vi "Andor Ixon_Settings.vi"() -> ()   [LabVIEW 2012]
uses:
  <userlib>/atmcd64d.llb/HSSpeed_type typedef.ctl
panel:
  in  "OK Button":bool
  in  "Vertical clock voltage":i32(ring) items=["Normal", "+1", "+2", "+3", "+4"]
  in  "Shift speed":i32(ring) items=["0.564720", "1.016496", "1.920048", "[3.727152]"]
  in  "Readout rate":i32(ring) items=["35.00MHz", "27.00MHz", "13.00MHz"]
  in  "Pre-amplifier gain":i32(ring) items=["1.000000x", "1.900000x", "3.700000x"]
  in  "Binning":i32[](array[numeric])
  in  "ROI":i32[][](array[numeric])
  in  "EM Gain":i32 min=3
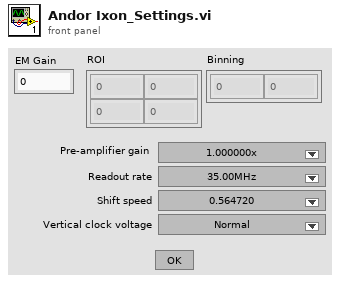
[diagram p1: front panel]
types:
  T1 = typedef "HSSpeed_type typedef.ctl" = enum16{"EM Amp", "Conventional Amp"}
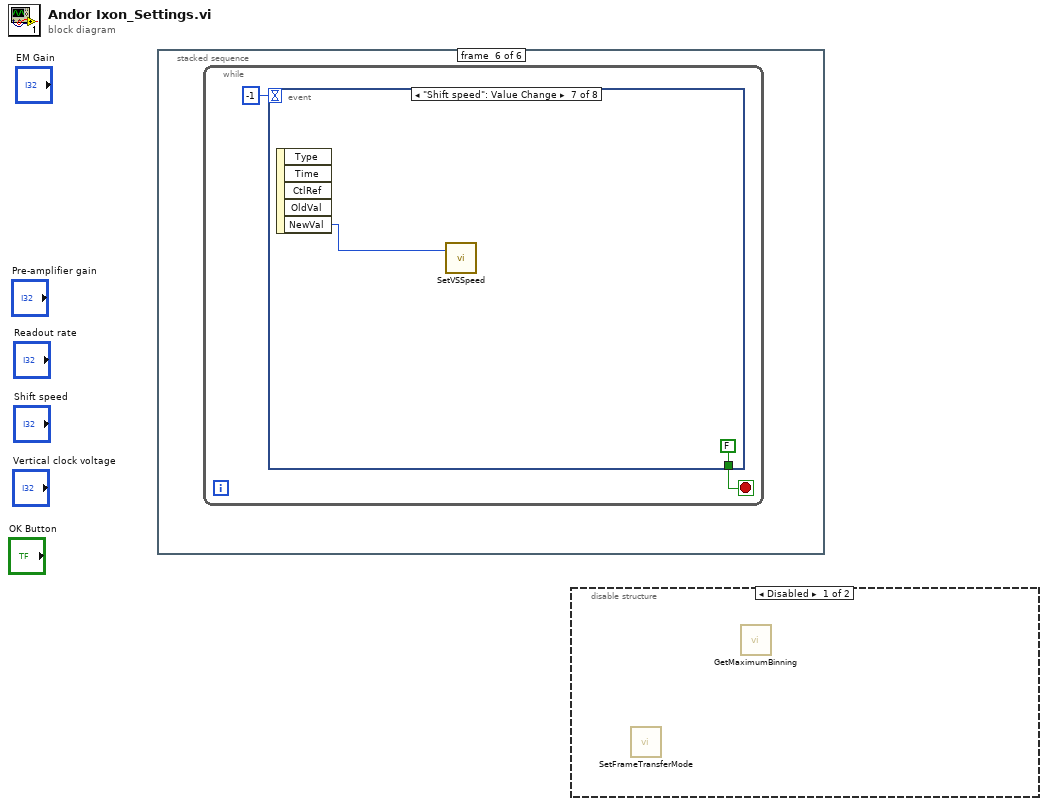
[diagram p0: block diagram]
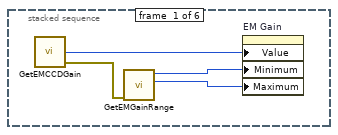
[diagram p3: hidden frame]
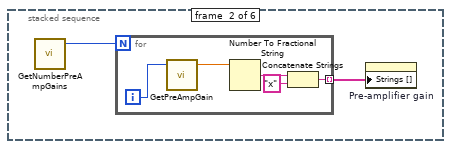
[diagram p4: hidden frame]
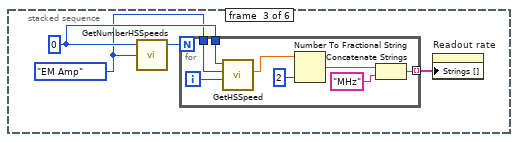
[diagram p5: hidden frame]
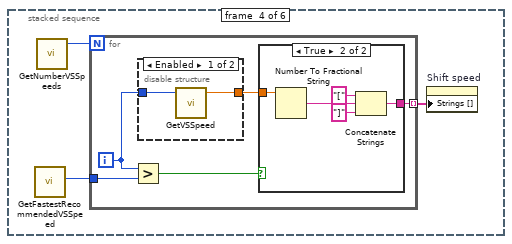
[diagram p6: hidden frame]
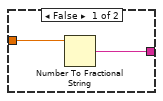
[diagram p7: hidden frame]
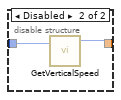
[diagram p8: hidden frame]
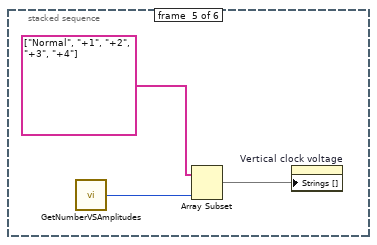
[diagram p9: hidden frame]
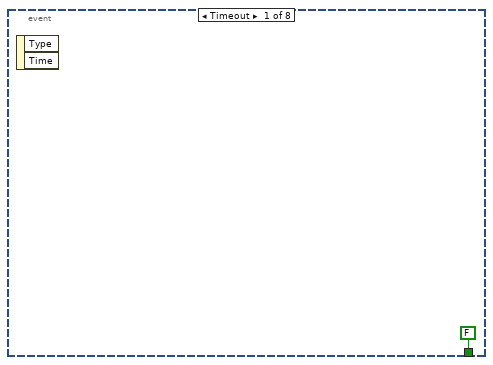
[diagram p10: hidden frame]
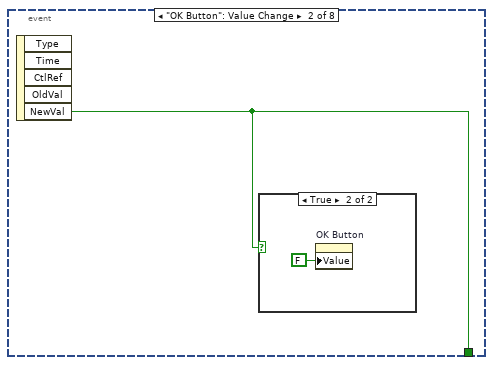
[diagram p11: hidden frame]
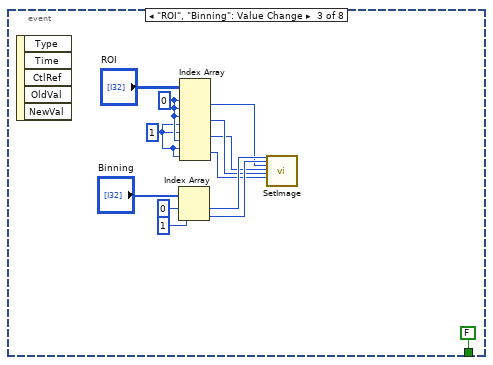
[diagram p13: hidden frame]
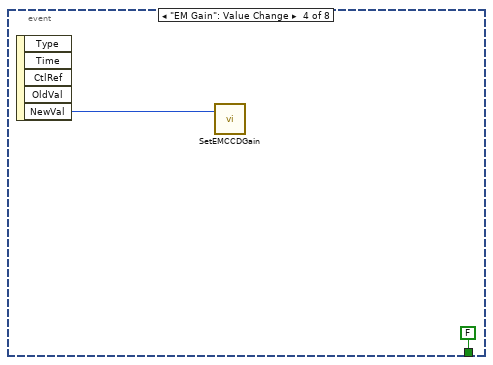
[diagram p14: hidden frame]
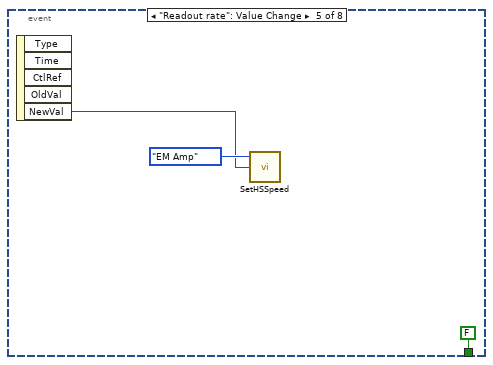
[diagram p15: hidden frame]
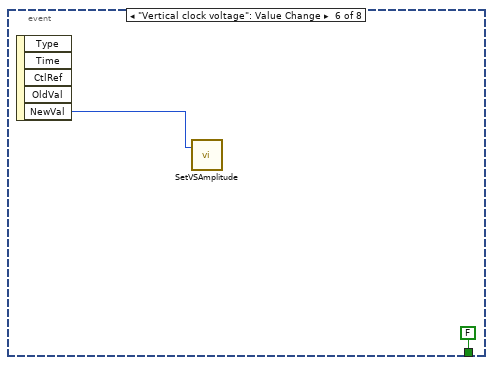
[diagram p16: hidden frame]
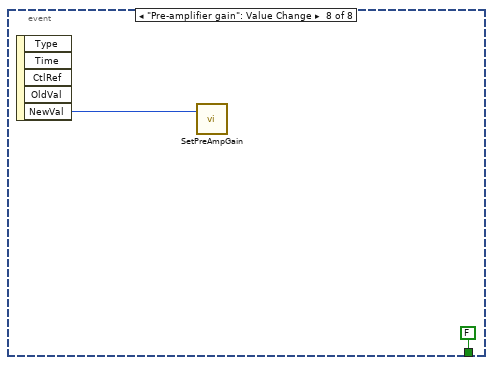
[diagram p17: hidden frame]
diagram:
  n1 = stacked-sequence {
    frame #0 {
      n2 = call <userlib>:"GetEMCCDGain.vi"() -> ("error out"=w1:errorcluster, "gain"=w4:u32)  [unwired: 3 in, 1 out]
      n3 = call <userlib>:"GetEMGainRange.vi"("error in (no error)"=w1) -> ("high"=w2:i32, "low"=w3:i32)  [unwired: 3 in, 2 out]
      n4 = property on="EM Gain" class="DigNum (strict)"("Value"=w4, "Minimum"=w3, "Maximum"=w2) -> ()  [unwired: 2 in, 2 out]
    }
    frame #1 {
      n5 = call <userlib>:"GetNumberPreAmpGains.vi"() -> ("number"=w5:i32)  [unwired: 3 in, 2 out]
      n6 = for {
        N: w5 -> [_]
        tunnel: [w9] -> w6 mode=indexing
        i -> [w8]
        n7 = call <userlib>:"GetPreAmpGain.vi"("index"=w8) -> ("gain"=w7:sgl)  [unwired: 2 in, 2 out]
        n8 = Number To Fractional String(number=w7) -> (F-format string=w11:string)  [unwired: 3 in]
        n9 = Concatenate Strings(w11, "x" ("string")) -> (w9:string)
      }
      n10 = property on="Pre-amplifier gain" class="Ring (strict)"("Strings []"=w6) -> ()  [unwired: 2 in, 2 out]
    }
    frame #2 {
      w12 = HSSpeed_type_typedef."EM Amp" ("type")
      w13 = 0 ("channel")
      n11 = call <userlib>:"GetNumberHSSpeeds.vi"("type"=w12, "channel"=w13) -> ("number"=w14:i32)  [unwired: 1 in, 2 out]
      n12 = for {
        N: w14 -> [_]
        tunnel: [w21] -> w15 mode=indexing
        tunnel: w13 -> [w18]
        tunnel: w12 -> [w17]
        i -> [w19]
        n13 = call <userlib>:"GetHSSpeed.vi"("index"=w19, "type"=w17, "channel"=w18) -> ("speed"=w20:sgl)  [unwired: 2 in, 2 out]
        n14 = Number To Fractional String(number=w20, precision (6)=i16 2) -> (F-format string=w23:string)  [unwired: 2 in]
        n15 = Concatenate Strings(w23, "MHz" ("string")) -> (w21:string)
      }
      n16 = property on="Readout rate" class="Ring (strict)"("Strings []"=w15) -> ()  [unwired: 2 in, 2 out]
    }
    frame #3 {
      n17 = call <userlib>:"GetFastestRecommendedVSSpeed.vi"() -> ("index"=w24:u32)  [unwired: 4 in, 3 out]
      n18 = call <userlib>:"GetNumberVSSpeeds.vi"() -> ("number"=w25:i32)  [unwired: 3 in, 2 out]
      n19 = for {
        N: w25 -> [_]
        tunnel: [w30] -> w26 mode=indexing
        tunnel: w24 -> [w28]
        i -> [w29]
        n20 = Greater?(x=w29, y=w28) -> (0:w27:bool)
        n21 = disable-structure shown="Enabled" {
          disable-tunnel: [w39 w41] -> w31
          disable-tunnel: w29 -> [w40 w42]
          frame Enabled {
            n22 = call <userlib>:"GetVSSpeed.vi"("index"=w40) -> ("speed"=w39:sgl)  [unwired: 2 in, 2 out]
          }
          frame Disabled {
            n23 = call <userlib>:"GetVerticalSpeed.vi"("index"=w42) -> ("speed"=w41:i32)  [unwired: 1 in, 2 out]
          }
        }
        n24 = case shown="True" w27 {
          tunnel: w31 -> [w33 w38]
          tunnel: [w32 w36] -> w30
          frame False {
            n25 = Number To Fractional String(number=w33) -> (F-format string=w32:string)  [unwired: 3 in]
          }
          frame True {
            n26 = Number To Fractional String(number=w38) -> (F-format string=w37:string)  [unwired: 3 in]
            n27 = Concatenate Strings("[" ("string"), w37, "]" ("string")) -> (w36:string)
          }
        }
      }
      n28 = property on="Shift speed" class="Ring (strict)"("Strings []"=w26) -> ()  [unwired: 2 in, 2 out]
    }
    frame #4 {
      n29 = call <userlib>:"GetNumberVSAmplitudes.vi"() -> ("number"=w43:i32)  [unwired: 3 in, 2 out]
      n30 = Array Subset(array=string[] ["Normal", "+1", "+2", "+3", "+4"], length=w43) -> (w44:string[])  [unwired: 1 in]
      n31 = property on="Vertical clock voltage" class="Ring (strict)"("Strings []"=w44) -> ()  [unwired: 2 in, 2 out]
    }
    frame #5 {
      n32 = while {
        stop <- w46 stop-if-true
        n33 = event shown="[6] \"Shift speed\": Value Change" {
          selector: _ -> [_ _ _ _ _ _ _ _]
          dyn-events: _ -> [_ _ _ _ _ _ _ _]
          timeout: -1 -> [_ _ _ _ _ _ _ _]
          tunnel: [FALSE ("NewVal") w49 FALSE ("NewVal") FALSE ("NewVal") FALSE ("NewVal") FALSE ("NewVal") FALSE ("NewVal") FALSE ("NewVal")] -> w46
          event Timeout {
            n34 = event-data() -> ()  [unwired: 1 in, 2 out]
          }
          event "OK Button": Value Change {
            n35 = event-data() -> ("NewVal"=w49:bool)  [unwired: 1 in, 4 out]
            n36 = case shown="True" w49 {
              frame False {
              }
              frame True {
                n37 = property on="OK Button" class="Bool (strict)"("Value"=FALSE ("OK Button")) -> ()  [unwired: 2 in, 2 out]
              }
            }
          }
          event "ROI", "Binning": Value Change {
            w55 = 1 ("index (row)")
            w56 = 0 ("index (row)")
            n38 = event-data() -> ()  [unwired: 1 in, 5 out]
            n39 = Index Array(array="Binning", index #1=0 ("index"), index #2=1 ("index")) -> (element #1=w61:i32, element #2=w58:i32)
            n40 = Index Array(array="ROI", index (row) #1=w56, index (col) #1=w56, index (row) #2=w56, index (col) #2=w55, index (row) #3=w55, index (col) #3=w56, index (row) #4=w55, index (col) #4=w55) -> (element #1=w54:i32, element #2=w53:i32, element #3=w51:i32, element #4=w52:i32)
            n41 = call <userlib>:"SetImage.vi"("hbin"=w61, "vbin"=w58, "hstart"=w54, "hend"=w51, "vstart"=w53, "vend"=w52) -> ()  [unwired: 20 in, 2 out]
          }
          event "EM Gain": Value Change {
            n42 = event-data() -> ("NewVal"=w64:i32)  [unwired: 1 in, 4 out]
            n43 = call <userlib>:"SetEMCCDGain.vi"("gain"=w64) -> ()  [unwired: 1 in, 2 out]
          }
          event "Readout rate": Value Change {
            n44 = event-data() -> ("NewVal"=w67:i32)  [unwired: 1 in, 4 out]
            n45 = call <userlib>:"SetHSSpeed.vi"("index"=w67, "type"=HSSpeed_type_typedef."EM Amp") -> ()  [unwired: 2 in, 2 out]
          }
          event "Vertical clock voltage": Value Change {
            n46 = event-data() -> ("NewVal"=w70:i32)  [unwired: 1 in, 4 out]
            n47 = call <userlib>:"SetVSAmplitude.vi"("amplitude"=w70) -> ()  [unwired: 1 in, 2 out]
          }
          event "Shift speed": Value Change {
            n48 = event-data() -> ("NewVal"=w72:i32)  [unwired: 1 in, 4 out]
            n49 = call <userlib>:"SetVSSpeed.vi"("index"=w72) -> ()  [unwired: 1 in, 2 out]
          }
          event "Pre-amplifier gain": Value Change {
            n50 = event-data() -> ("NewVal"=w74:i32)  [unwired: 1 in, 4 out]
            n51 = call <userlib>:"SetPreAmpGain.vi"("index"=w74) -> ()  [unwired: 1 in, 2 out]
          }
        }
      }
    }
  }
  n52 = disable-structure shown="Disabled" {
    frame Disabled {
      n53 = call <userlib>:"SetFrameTransferMode.vi"() -> ()  [unwired: 2 in, 2 out]
      n54 = call <userlib>:"GetMaximumBinning.vi"() -> ()  [unwired: 3 in, 3 out]
    }
    frame Enabled {
    }
  }
